vi "XYZ stage communication_MD.vi"   [LabVIEW 2012]
uses:
  <vilib>/Utility/VariantDataType/Type.ctl
  GFG/GFGstringGet.vi
  <vilib>/Instr/_visa.llb/VISA Configure Serial Port (Instr).vi
  GFG/GFGnumericGet.vi
  GFG/GFGbooleanGet.vi
  GFG/GFG library.lvlib
  <vilib>/Utility/VariantDataType/VariantType.lvlib
types:
  T1 = cluster{"moveXabs":dbl, "moveYabs":dbl, "moveZabs":dbl}
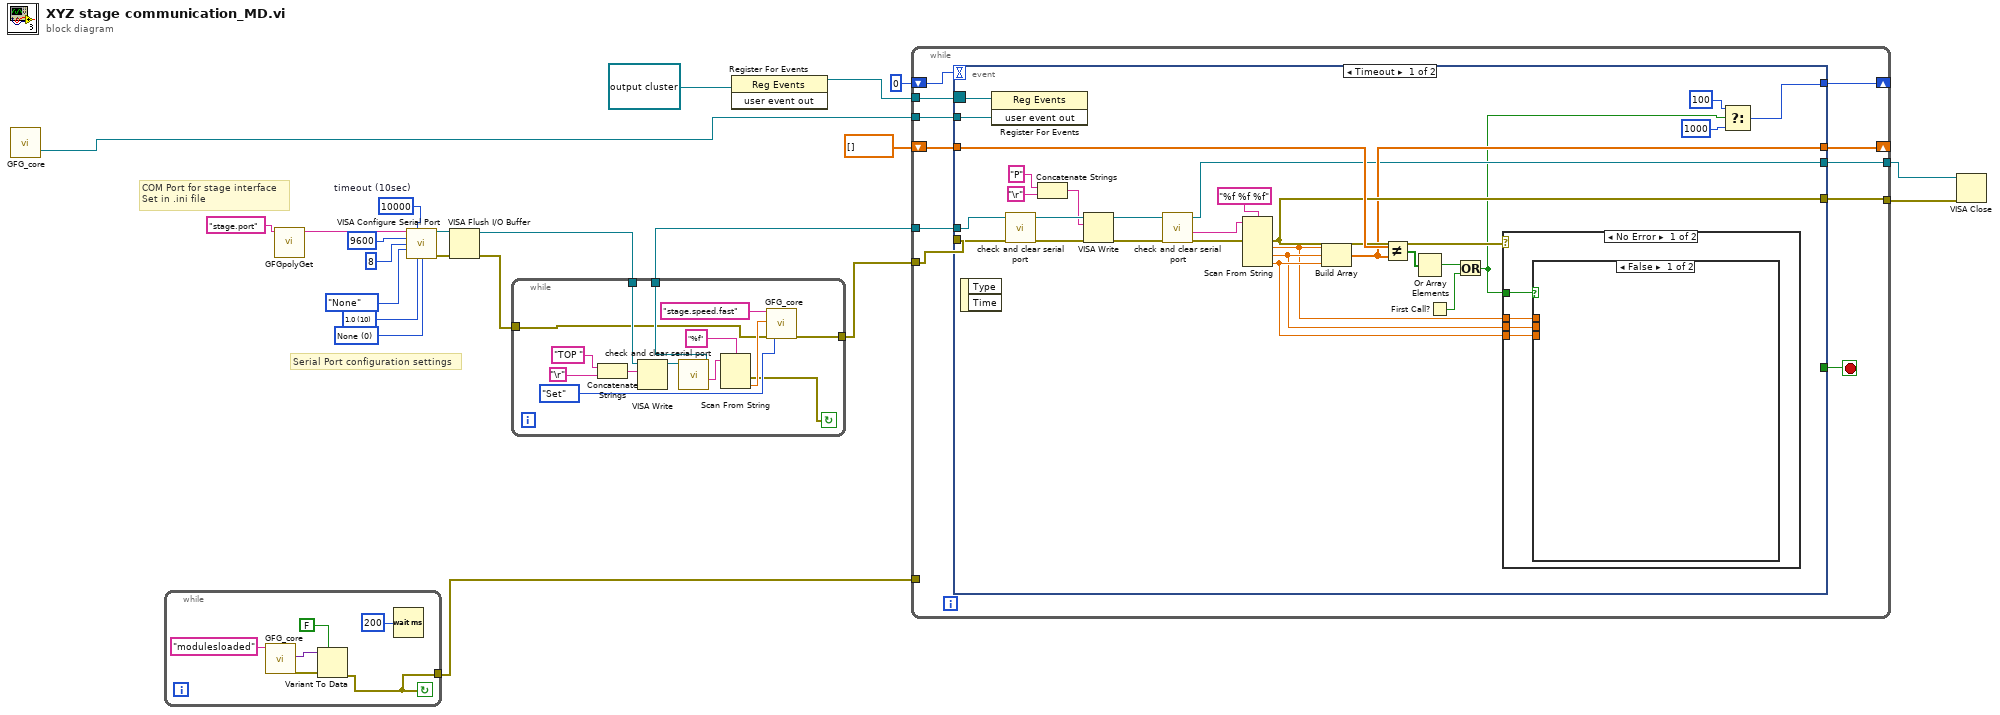
[diagram p0: block diagram]
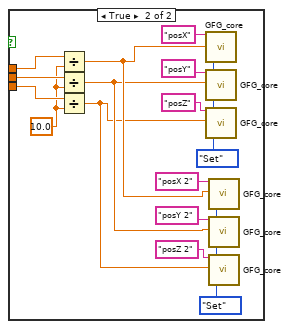
[diagram p2: hidden frame]
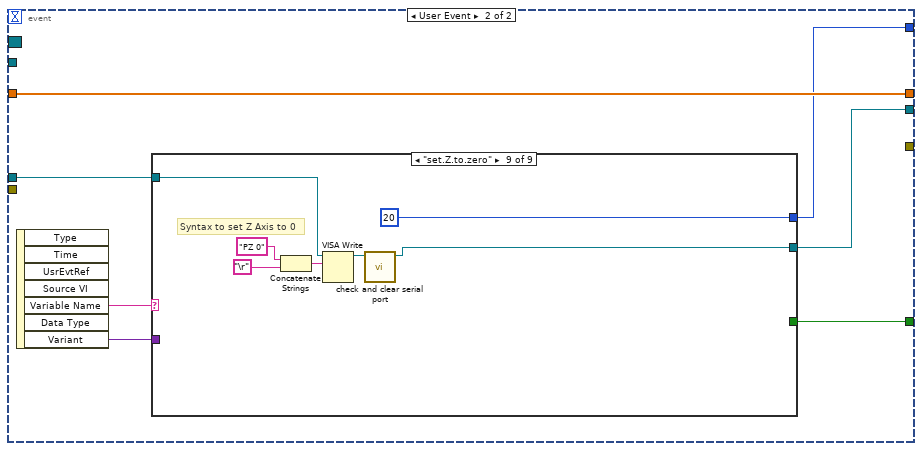
[diagram p4: hidden frame]
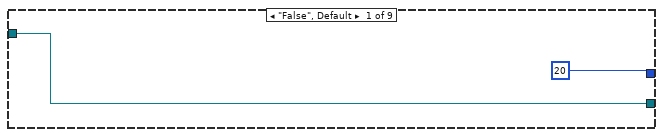
[diagram p5: hidden frame]
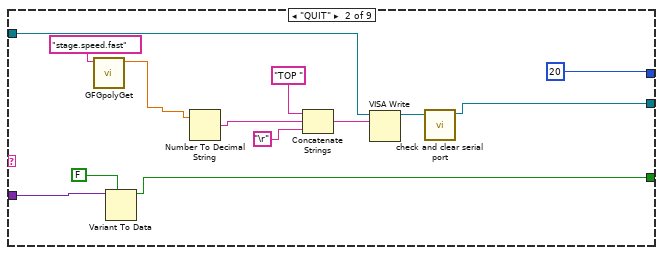
[diagram p6: hidden frame]
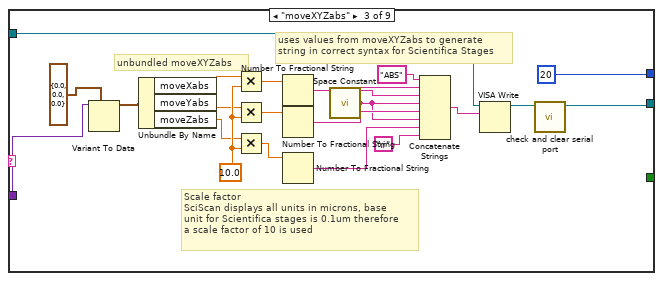
[diagram p7: hidden frame]
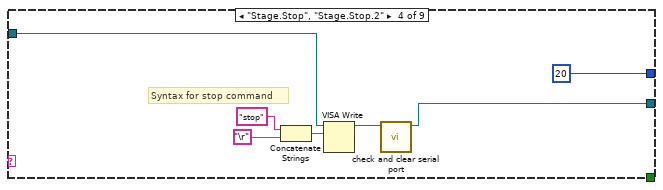
[diagram p8: hidden frame]
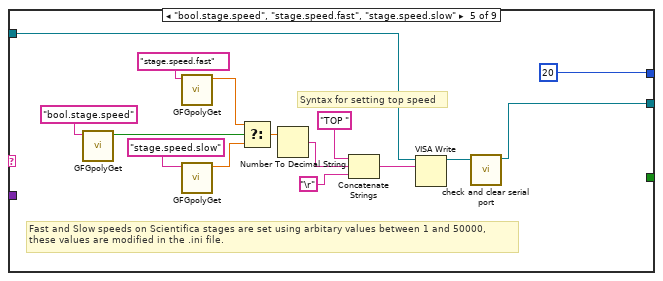
[diagram p9: hidden frame]
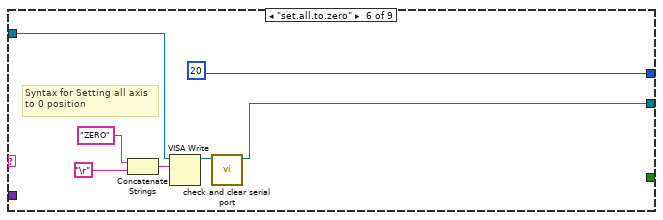
[diagram p10: hidden frame]
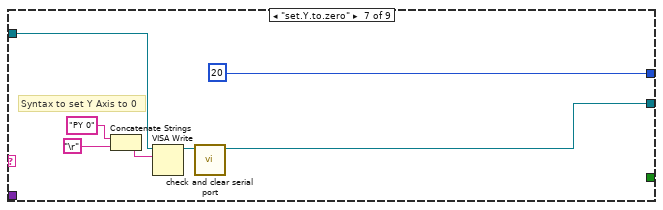
[diagram p11: hidden frame]
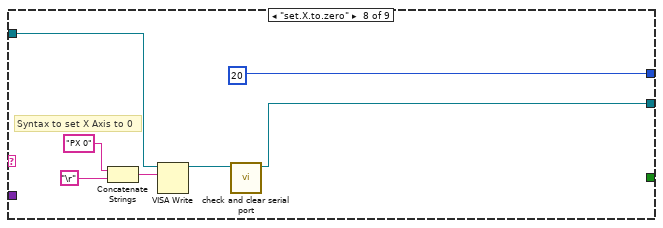
[diagram p12: hidden frame]
diagram:
  w15 = u16 0 items=["None", "XON/XOFF", "RTS/CTS", "XON/XOFF & RTS/CTS", "DTR/DSR", "XON/XOFF & DTR/DSR"] ("flow control (0:none)")
  w16 = u16 10 items=["1.0"=10, "1.5"=15, "2.0"=20] ("stop bits (10: 1 bit)")
  w20 = u32 10000  # timeout (10sec)
  # "COM Port for stage interface\nSet in .ini file"
  # "Serial Port configuration settings"
  n1 = call "GFG_core.vi"() -> ("user event out"=w3:refnum<user-event>)  [unwired: 13 in, 6 out]
  n2 = while {
    tunnel: [w23] -> w1
    stop <- w23 continue-if-true
    n3 = call "GFG_core.vi"("Variable Name in"="modulesloaded") -> ("Variant Out"=w24:variant, "error out"=w26:errorcluster)  [unwired: 12 in, 5 out]
    n4 = Variant To Data(error in=w26, type=FALSE, Variant=w24) -> (error out=w23:errorcluster)  [unwired: 1 out]
    n5 = Wait (ms)(milliseconds to wait=u32 200) -> ()  [unwired: 1 out]
  }
  n6 = call-poly "GFGpolyGet.vi"("Variable Name in"="stage.port") -> ("String"=w12:string)  [unwired: 10 in]
  n7 = call-poly "VISA Configure Serial Port"("VISA resource name"=w12, "timeout (10sec)"=w20, "baud rate (9600)"=u32 9600, "data bits (8)"=u16 8, "parity (0:none)"=enum16{"None", "Odd", "Even", "Mark", "Space"}."None", "stop bits (10: 1 bit)"=w16, "flow control (0:none)"=w15) -> ("VISA resource name out"=w14:refnum<visa-resource-name>, "error out"=w13:errorcluster)  [unwired: 7 in]
  n8 = VISA Flush I/O Buffer(VISA resource name=w14, error in (no error)=w13) -> (VISA resource name out=w6:refnum<visa-resource-name>, error out=w4:errorcluster)  [unwired: 1 in]
  n9 = while {
    tunnel: w6 -> [w38]
    tunnel: [w37] -> w5
    tunnel: w4 -> [w30]
    tunnel: [w29] -> w2
    stop <- w31 continue-if-true
    n10 = Concatenate Strings("TOP " ("write buffer"), "\r") -> (w41:string)
    n11 = VISA Write(VISA resource name=w38, write buffer=w41) -> (VISA resource name out=w40:refnum<visa-resource-name>)  [unwired: 1 in, 2 out]
    n12 = call "check and clear serial port.vi"("VISA resource name in"=w40) -> ("read buffer"=w33:string, "VISA resource name out"=w37:refnum<visa-resource-name>)  [unwired: 7 in, 2 out]
    n13 = Scan From String(format string="%f", input string=w33) -> (error out=w31:errorcluster, output 1=w32:dbl)  [unwired: 3 in, 2 out]
    n14 = call "GFG_core.vi"("Variable Name in"="stage.speed.fast", "Variant in"=w32, "error in (no error)"=w30, "Action"=enum16{"Init", "Set", "Get"}."Set") -> ("error out"=w29:errorcluster)  [unwired: 9 in, 6 out]
  }
  n15 = register-events(refnum<user-event> refnum ("user event out")) -> (reference out=w7:refnum<event-registration>)  [unwired: 2 in, 1 out]
  n16 = while {
    tunnel: [w53] -> w10
    tunnel: w5 -> [w52]
    shift-right: [w51] -> _
    shift-left: dbl[] [] -> [w49]
    tunnel: [w48] -> w9
    shift-right: [w46] -> _
    shift-left: 0 -> [w47]
    tunnel: w3 -> [w45]
    tunnel: w7 -> [w44]
    tunnel: w2 -> [w43]
    tunnel: w1 -> [_]
    stop <- w50 stop-if-true
    n17 = event shown="[0] Timeout" {
      selector: w44 -> [w58 _]
      dyn-events: _ -> [_ _]
      timeout: w47 -> [_ _]
      tunnel: [w67 w103] -> w53
      tunnel: w52 -> [w76 w104]
      tunnel: [w79 w102] -> w51
      tunnel: [_ w105] -> w50
      tunnel: w49 -> [w81 w102]
      tunnel: w43 -> [w74 _]
      tunnel: [w80 _] -> w48
      tunnel: [w61 w101] -> w46
      tunnel: w45 -> [w57 _]
      event Timeout {
        n18 = event-data() -> ()  [unwired: 1 in, 2 out]
        n19 = register-events(reference=w58, w57) -> ()  [unwired: 1 in, 2 out]
        n20 = call "check and clear serial port.vi"("error in (no error)"=w74, "VISA resource name in"=w76) -> ("error out"=w73:errorcluster, "VISA resource name out"=w75:refnum<visa-resource-name>)  [unwired: 6 in, 2 out]
        n21 = Concatenate Strings("P" ("write buffer"), "\r") -> (w65:string)
        n22 = VISA Write(VISA resource name=w75, write buffer=w65, error in (no error)=w73) -> (VISA resource name out=w69:refnum<visa-resource-name>, error out=w70:errorcluster)  [unwired: 1 out]
        n23 = call "check and clear serial port.vi"("error in (no error)"=w70, "VISA resource name in"=w69) -> ("error out"=w68:errorcluster, "read buffer"=w66:string, "VISA resource name out"=w67:refnum<visa-resource-name>)  [unwired: 6 in, 1 out]
        n24 = Scan From String(format string="%f %f %f", input string=w66, error in=w68) -> (error out=w80:errorcluster, output 1=w54:dbl, output 2=w55:dbl, output 3=w56:dbl)  [unwired: 4 in, 2 out]
        n25 = Build Array(w54, w55, w56) -> (w79:dbl[])
        n26 = Not Equal?(x=w81, y=w79) -> (x != y?=w78:bool[])
        n27 = Or Array Elements(Boolean array=w78) -> (logical OR=w62:bool)
        n28 = First Call?() -> (First Call?: T/F=w60:bool)
        n29 = Or(x=w62, y=w60) -> (x .or. y?=w59:bool)
        n30 = case shown="No Error" w80 {
          tunnel: w54 -> [w83 _]
          tunnel: w55 -> [w84 _]
          tunnel: w56 -> [w85 _]
          tunnel: w59 -> [w82 _]
          frame No Error {
            n31 = case shown="False" w82 {
              tunnel: w85 -> [_ w97]
              tunnel: w84 -> [_ w96]
              tunnel: w83 -> [_ w95]
              frame False {
              }
              frame True {
                w92 = enum16{"Init", "Set", "Get"}."Set" ("Action")
                w94 = 10.0 ("y")
                w93 = enum16{"Init", "Set", "Get"}."Set" ("Action")
                n32 = Divide(x=w95, y=w94) -> (x/y=w88:dbl)
                n33 = Divide(x=w96, y=w94) -> (x/y=w87:dbl)
                n34 = Divide(x=w97, y=w94) -> (x/y=w86:dbl)
                n35 = call "GFG_core.vi"("Variable Name in"="posX", "Variant in"=w88, "Action"=w93) -> ()  [unwired: 10 in, 7 out]
                n36 = call "GFG_core.vi"("Variable Name in"="posY", "Variant in"=w87, "Action"=w93) -> ()  [unwired: 10 in, 7 out]
                n37 = call "GFG_core.vi"("Variable Name in"="posZ", "Variant in"=w86, "Action"=w93) -> ()  [unwired: 10 in, 7 out]
                n38 = call "GFG_core.vi"("Variable Name in"="posX 2", "Variant in"=w88, "Action"=w92) -> ()  [unwired: 10 in, 7 out]
                n39 = call "GFG_core.vi"("Variable Name in"="posY 2", "Variant in"=w87, "Action"=w92) -> ()  [unwired: 10 in, 7 out]
                n40 = call "GFG_core.vi"("Variable Name in"="posZ 2", "Variant in"=w86, "Action"=w92) -> ()  [unwired: 10 in, 7 out]
              }
            }
          }
          frame Error {
          }
        }
        n41 = Select(t=100, s=w59, f=1000) -> (s? t:f=w61:i32)
      }
      event User Event {
        n42 = event-data() -> ("Variable Name"=w107:string, "Variant"=w106:variant)  [unwired: 1 in, 5 out]
        n43 = case shown="\"set.Z.to.zero\"" w107 {
          tunnel: [_ w120 _ _ _ _ _ _ _] -> w105
          tunnel: w106 -> [_ w122 w128 _ _ _ _ _ _]
          tunnel: w104 -> [w109 w115 w138 w146 w153 w170 w177 w184 w193]
          tunnel: [w109 w114 w131 w145 w152 w168 w175 w182 w192] -> w103
          tunnel: [20 20 20 20 20 20 20 20 20] -> w101
          frame "False", Default {
          }
          frame "QUIT" {
            n44 = call-poly "GFGpolyGet.vi"("Variable Name in"="stage.speed.fast") -> ("Numeric"=w112:dbl)  [unwired: 9 in, 1 out]
            n45 = Variant To Data(type=FALSE ("NewVal"), Variant=w122) -> (data=w120:bool)  [unwired: 1 in, 1 out]
            n46 = Number To Decimal String(number=w112) -> (decimal integer string=w110:string)  [unwired: 1 in]
            n47 = Concatenate Strings("TOP " ("write buffer"), w110, "\r") -> (w117:string)
            n48 = VISA Write(VISA resource name=w115, write buffer=w117) -> (VISA resource name out=w118:refnum<visa-resource-name>)  [unwired: 1 in, 2 out]
            n49 = call "check and clear serial port.vi"("VISA resource name in"=w118) -> ("VISA resource name out"=w114:refnum<visa-resource-name>)  [unwired: 7 in, 3 out]
          }
          frame "moveXYZabs" {
            w133 = 10.0 ("y")
            # "Scale factor \nSciScan displays all units in microns, base \nunit for Scientifica stages is 0.1um therefore \na scale factor of 10 is used"
            # "unbundled moveXYZabs"
            # "uses values from moveXYZabs to generate\nstring in correct syntax for Scientifica Stages"
            n50 = Variant To Data(type=T1 {"moveXabs"=0.0, "moveYabs"=0.0, "moveZabs"=0.0} ("output cluster"), Variant=w128) -> (data=w126:T1)  [unwired: 1 in, 1 out]
            n51 = Unbundle By Name(w126) -> ("moveXabs"=w123:dbl, "moveYabs"=w124:dbl, "moveZabs"=w125:dbl)
            n52 = Multiply(x=w123, y=w133) -> (x*y=w136:dbl)
            n53 = Multiply(x=w124, y=w133) -> (x*y=w135:dbl)
            n54 = Multiply(x=w125, y=w133) -> (x*y=w134:dbl)
            n55 = Number To Fractional String(number=w136) -> (F-format string=w143:string)  [unwired: 3 in]
            n56 = Number To Fractional String(number=w135) -> (F-format string=w142:string)  [unwired: 3 in]
            n57 = Number To Fractional String(number=w134) -> (F-format string=w141:string)  [unwired: 3 in]
            n58 = call <vilib>:"Space Constant.vi"() -> ("String"=w140:string)
            n59 = Concatenate Strings("ABS" ("string"), w140, w143, w140, w142, w140, w141, "\r") -> (w130:string)
            n60 = VISA Write(VISA resource name=w138, write buffer=w130) -> (VISA resource name out=w132:refnum<visa-resource-name>)  [unwired: 1 in, 2 out]
            n61 = call "check and clear serial port.vi"("VISA resource name in"=w132) -> ("VISA resource name out"=w131:refnum<visa-resource-name>)  [unwired: 7 in, 3 out]
          }
          frame "Stage.Stop", "Stage.Stop.2" {
            # "Syntax for stop command"
            n62 = Concatenate Strings("stop" ("write buffer"), "\r") -> (w150:string)
            n63 = VISA Write(VISA resource name=w146, write buffer=w150) -> (VISA resource name out=w149:refnum<visa-resource-name>)  [unwired: 1 in, 2 out]
            n64 = call "check and clear serial port.vi"("VISA resource name in"=w149) -> ("VISA resource name out"=w145:refnum<visa-resource-name>)  [unwired: 7 in, 3 out]
          }
          frame "bool.stage.speed", "stage.speed.fast", "stage.speed.slow" {
            # "Syntax for setting top speed"
            # "Fast and Slow speeds on Scientifica stages are set using arbitary values between 1 and 50000, \nthese values are modified in the .ini file."
            n65 = call-poly "GFGpolyGet.vi"("Variable Name in"="bool.stage.speed") -> ("Boolean"=w156:bool)  [unwired: 10 in]
            n66 = call-poly "GFGpolyGet.vi"("Variable Name in"="stage.speed.fast") -> ("Numeric"=w158:dbl)  [unwired: 9 in, 1 out]
            n67 = call-poly "GFGpolyGet.vi"("Variable Name in"="stage.speed.slow") -> ("Numeric"=w157:dbl)  [unwired: 9 in, 1 out]
            n68 = Select(t=w158, s=w156, f=w157) -> (s? t:f=w155:dbl)
            n69 = Number To Decimal String(number=w155) -> (decimal integer string=w154:string)  [unwired: 1 in]
            n70 = Concatenate Strings("TOP " ("write buffer"), w154, "\r") -> (w164:string)
            n71 = VISA Write(VISA resource name=w153, write buffer=w164) -> (VISA resource name out=w165:refnum<visa-resource-name>)  [unwired: 1 in, 2 out]
            n72 = call "check and clear serial port.vi"("VISA resource name in"=w165) -> ("VISA resource name out"=w152:refnum<visa-resource-name>)  [unwired: 7 in, 3 out]
          }
          frame "set.all.to.zero" {
            # "Syntax for Setting all axis \nto 0 position"
            n73 = Concatenate Strings("ZERO" ("write buffer"), "\r") -> (w166:string)
            n74 = VISA Write(VISA resource name=w170, write buffer=w166) -> (VISA resource name out=w169:refnum<visa-resource-name>)  [unwired: 1 in, 2 out]
            n75 = call "check and clear serial port.vi"("VISA resource name in"=w169) -> ("VISA resource name out"=w168:refnum<visa-resource-name>)  [unwired: 7 in, 3 out]
          }
          frame "set.Y.to.zero" {
            # "Syntax to set Y Axis to 0"
            n76 = Concatenate Strings("PY 0" ("write buffer"), "\r") -> (w174:string)
            n77 = VISA Write(VISA resource name=w177, write buffer=w174) -> (VISA resource name out=w176:refnum<visa-resource-name>)  [unwired: 1 in, 2 out]
            n78 = call "check and clear serial port.vi"("VISA resource name in"=w176) -> ("VISA resource name out"=w175:refnum<visa-resource-name>)  [unwired: 7 in, 3 out]
          }
          frame "set.X.to.zero" {
            # "Syntax to set X Axis to 0"
            n79 = Concatenate Strings("PX 0" ("write buffer"), "\r") -> (w181:string)
            n80 = VISA Write(VISA resource name=w184, write buffer=w181) -> (VISA resource name out=w183:refnum<visa-resource-name>)  [unwired: 1 in, 2 out]
            n81 = call "check and clear serial port.vi"("VISA resource name in"=w183) -> ("VISA resource name out"=w182:refnum<visa-resource-name>)  [unwired: 7 in, 3 out]
          }
          frame "set.Z.to.zero" {
            # "Syntax to set Z Axis to 0"
            n82 = Concatenate Strings("PZ 0" ("write buffer"), "\r") -> (w187:string)
            n83 = VISA Write(VISA resource name=w193, write buffer=w187) -> (VISA resource name out=w188:refnum<visa-resource-name>)  [unwired: 1 in, 2 out]
            n84 = call "check and clear serial port.vi"("VISA resource name in"=w188) -> ("VISA resource name out"=w192:refnum<visa-resource-name>)  [unwired: 7 in, 3 out]
          }
        }
      }
    }
  }
  n85 = VISA Close(VISA resource name=w10, error in (no error)=w9) -> ()  [unwired: 1 out]
